vi "Main_PWM.vi"() -> ()   [LabVIEW 2015]
doc: "View output from heater including temperature, heater status, temp set point, heater set, and current PWM output (as controlled by PID)."
uses:
  <vilib>/Instr/_visa.llb/VISA Configure Serial Port (Instr).vi
panel:
  out "PWM":i32
  out "On/Off Set":bool
  out "Measurement History":waveform(dbl)(graph)
  out "Set Point FB":i32 caption="Temp Set Point (C)"
  out "Heater Status":bool
  out "Temp (C)":dbl
  in  "Set Point (C)":i32 caption="Temp Set Point (C)" min=0 max=40
  in  "Heater":bool
  in  "String":string
  in  "Send":bool
  in  "stop":bool
  out "Time of Read":string
  out "Serial Buffer":string
  in  "VISA resource name":refnum<visa-resource-name>
  # "Fluid Heater Control"
  # "Feedback"
  # "Setpoint"
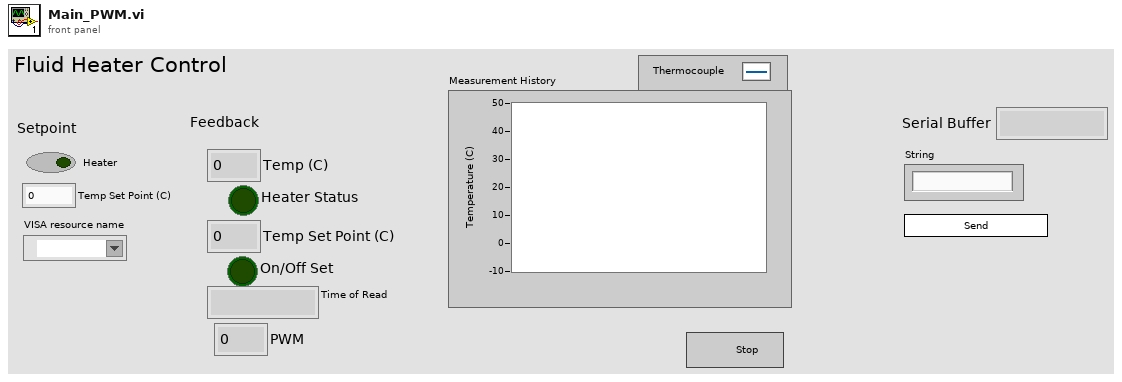
[diagram p1: front panel]
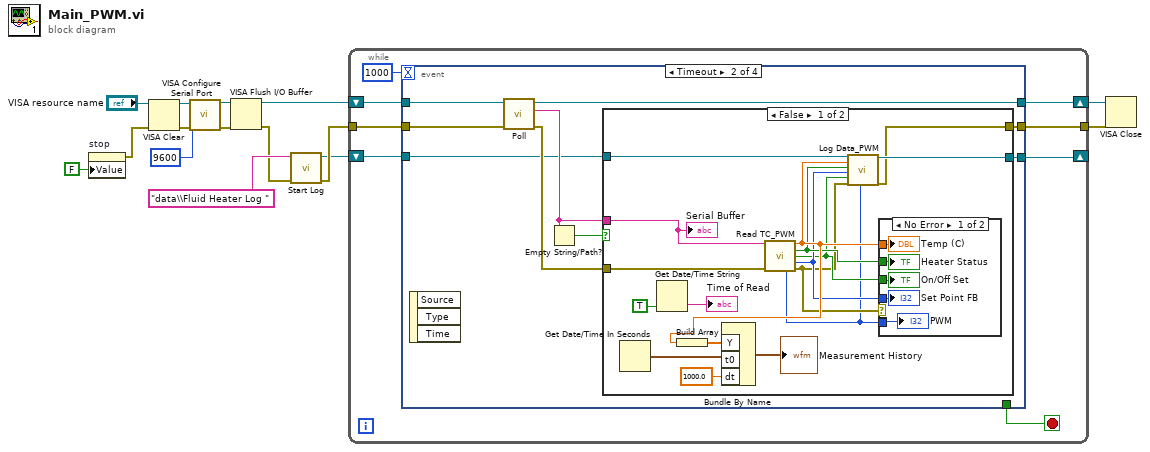
[diagram p0: block diagram]
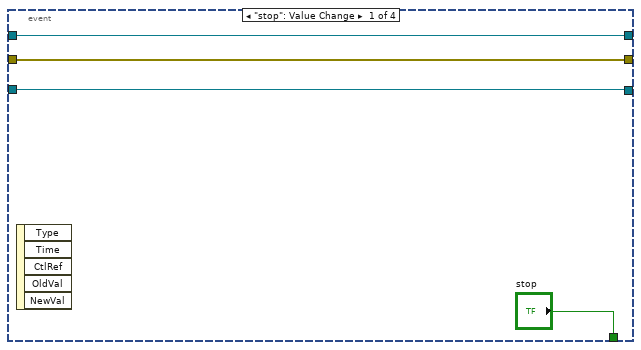
[diagram p2: hidden frame]
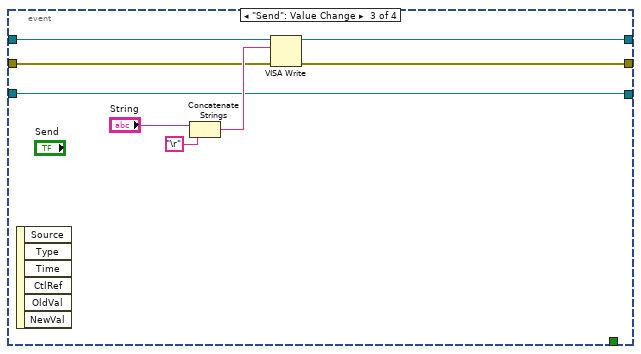
[diagram p5: hidden frame]
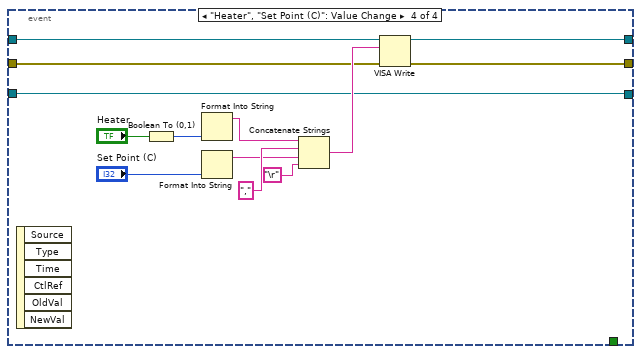
[diagram p6: hidden frame]
diagram:
  n1 = property on="stop" class="Bool (strict)"("Value"=FALSE ("stop")) -> (error out=w6:errorcluster)  [unwired: 2 in, 1 out]
  n2 = VISA Clear(VISA resource name="VISA resource name", error in (no error)=w6) -> (VISA resource name out=w11:refnum<visa-resource-name>, error out=w14:errorcluster)
  n3 = call-poly "VISA Configure Serial Port"("VISA resource name"=w11, "baud rate (9600)"=u32 9600, "error in (no error)"=w14) -> ("VISA resource name out"=w10:refnum<visa-resource-name>, "error out"=w15:errorcluster)  [unwired: 11 in]
  n4 = VISA Flush I/O Buffer(VISA resource name=w10, error in (no error)=w15) -> (VISA resource name out=w9:refnum<visa-resource-name>, error out=w3:errorcluster)  [unwired: 1 in]
  n5 = call "Start Log.vi"("Error In"=w3, "Log Prefix"="data\\Fluid Heater Log ") -> ("Error Out"=w2:errorcluster, "refnum out"=w1:refnum<file>)  [unwired: 8 in]
  n6 = while {
    tunnel: w2 -> [w20]
    shift-right: [w19] -> w8
    shift-left: w9 -> [w21]
    tunnel: [w18] -> w7
    shift-right: [w16] -> _
    shift-left: w1 -> [w17]
    stop <- w23 stop-if-true
    n7 = event shown="[1] Timeout" {
      selector: _ -> [_ _ _ _]
      dyn-events: _ -> [_ _ _ _]
      timeout: 1000 -> [_ _ _ _]
      tunnel: ["stop" _ _ _] -> w23
      tunnel: w21 -> [w26 w34 w65 w73]
      tunnel: w20 -> [w25 w33 w63 w72]
      tunnel: [w26 w32 w64 w71] -> w19
      tunnel: [w25 w28 w62 w70] -> w18
      tunnel: w17 -> [w24 w30 w61 w69]
      tunnel: [w24 w29 w61 w69] -> w16
      event "stop": Value Change {
        n8 = event-data() -> ()  [unwired: 1 in, 5 out]
      }
      event Timeout {
        n9 = event-data() -> ()  [unwired: 1 in, 3 out]
        n10 = call "Poll.vi"("error in"=w33, "VISA resource name in"=w34) -> ("error out"=w31:errorcluster, "Read"=w36:string, "VISA resource name out"=w32:refnum<visa-resource-name>)  [unwired: 7 in]
        n11 = Empty String/Path?(string/path=w36) -> (empty?=w35:bool)
        n12 = case shown="False" w35 {
          tunnel: w36 -> [w51 _]
          tunnel: w31 -> [w50 w59]
          tunnel: w30 -> [w40 w60]
          tunnel: [w39 w60] -> w29
          tunnel: [w38 w59] -> w28
          frame False {
            n13 = Get Date/Time In Seconds() -> (seconds since 1Jan1904=w49:timestamp)
            n14 = Get Date/Time String(want seconds? (F)=TRUE) -> (time string=→"Time of Read":string)  [unwired: 2 in, 1 out]
            n15 = call "Read TC_PWM.vi"("read buffer"=w51, "Error In"=w50) -> ("Temp (C)"=w45:dbl, "On/Off Actual"=w44:bool, "On/Off Set"=w42:bool, "Temp Set Point (C)"=w43:i32, "PWM"=w37:i32, "Error Out"=w41:errorcluster)  [unwired: 8 in]
            n16 = Build Array(w45) -> (w48:dbl[])
            n17 = Bundle By Name("Y"=w48, "t0"=w49, "dt"=1000.0) -> (→"Measurement History":waveform(dbl))  [unwired: 1 in]
            n18 = call "Log Data_PWM.vi"("refnum in"=w40, "Temp (C)"=w45, "Heater Status"=w44, "Set Point FB"=w43, "On/Off Set"=w42, "Error In"=w41, "PWM"=w37) -> ("refnum out"=w39:refnum<file>, "Error Out"=w38:errorcluster)  [unwired: 11 in]
            n19 = case shown="No Error" w41 {
              tunnel: w45 -> [w58 _]
              tunnel: w44 -> [w57 _]
              tunnel: w43 -> [w56 _]
              tunnel: w42 -> [w55 _]
              tunnel: [w54 _] -> _
              tunnel: w37 -> [w54 _]
              frame No Error {
                "Temp (C)" <- w58
                "Heater Status" <- w57
                "Set Point FB" <- w56
                "On/Off Set" <- w55
                "PWM" <- w54
              }
              frame Error {
              }
            }
            "Serial Buffer" <- w51
          }
          frame True {
          }
        }
      }
      event "Send": Value Change {
        n20 = event-data() -> ()  [unwired: 1 in, 6 out]
        n21 = Concatenate Strings("String", "\r") -> (w66:string)
        n22 = VISA Write(VISA resource name=w65, write buffer=w66, error in (no error)=w63) -> (VISA resource name out=w64:refnum<visa-resource-name>, error out=w62:errorcluster)  [unwired: 1 out]
      }
      event "Heater", "Set Point (C)": Value Change {
        n23 = event-data() -> ()  [unwired: 1 in, 6 out]
        n24 = Boolean To (0,1)(Boolean="Heater") -> (0, 1=w77:i16)
        n25 = Format Into String(w77) -> (resulting string=w74:string)  [unwired: 3 in, 1 out]
        n26 = Format Into String("Set Point (C)") -> (resulting string=w75:string)  [unwired: 3 in, 1 out]
        n27 = Concatenate Strings(w74, ",", w75, "\r") -> (w80:string)
        n28 = VISA Write(VISA resource name=w73, write buffer=w80, error in (no error)=w72) -> (VISA resource name out=w71:refnum<visa-resource-name>, error out=w70:errorcluster)  [unwired: 1 out]
      }
    }
  }
  n29 = VISA Close(VISA resource name=w8, error in (no error)=w7) -> ()  [unwired: 1 out]
